vi "Start Async.vi"(8 "error in (no error)":errorcluster, 11 "gRPC Server in":refnum<class "dcvmDPI.lvclass">) -> (0 "error out":errorcluster, 3 "gRPC Server out":refnum<class "dcvmDPI.lvclass">)   [LabVIEW 2021, in "dcvmDPI_AD7606B_server.lvlib" / "dcvmDPI.lvclass"]
uses:
  dcvmDPI.lvclass
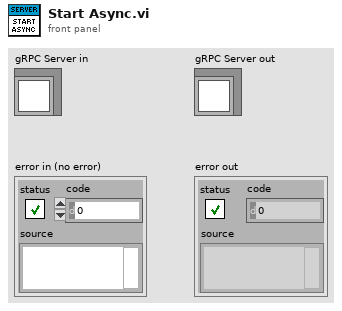
[diagram p1: front panel]
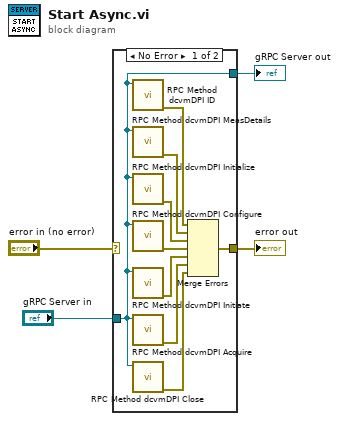
[diagram p0: block diagram]
diagram:
  n1 = case shown="No Error" "error in (no error)" {
    selector: "error in (no error)" -> [_ w15]
    tunnel: [w13 w15] -> w3
    tunnel: [w12 w14] -> w1
    tunnel: "gRPC Server in" -> [w12 w14]
    frame No Error {
      n2 = call "RPC Method dcvmDPI ID.vi"("OOP Server in"=w12) -> ("error out"=w11:errorcluster)  [unwired: 9 in, 1 out]
      n3 = call "RPC Method dcvmDPI MeasDetails.vi"("OOP Server in"=w12) -> ("error out"=w10:errorcluster)  [unwired: 9 in, 1 out]
      n4 = call "RPC Method dcvmDPI Initialize.vi"("OOP Server in"=w12) -> ("error out"=w9:errorcluster)  [unwired: 9 in, 1 out]
      n5 = call "RPC Method dcvmDPI Configure.vi"("OOP Server in"=w12) -> ("error out"=w8:errorcluster)  [unwired: 9 in, 1 out]
      n6 = call "RPC Method dcvmDPI Initiate.vi"("OOP Server in"=w12) -> ("error out"=w7:errorcluster)  [unwired: 9 in, 1 out]
      n7 = call "RPC Method dcvmDPI Acquire.vi"("OOP Server in"=w12) -> ("error out"=w6:errorcluster)  [unwired: 9 in, 1 out]
      n8 = call "RPC Method dcvmDPI Close.vi"("OOP Server in"=w12) -> ("error out"=w5:errorcluster)  [unwired: 9 in, 1 out]
      n9 = Merge Errors(w11, w10, w9, w8, w7, w6, w5) -> (w13:errorcluster)
    }
    frame Error {
    }
  }
  "error out" <- w3
  "gRPC Server out" <- w1
